vi "Pre Launch Init.vi"(11 "DIMActor in":refnum<class "DIMActor.lvclass">) -> (0 "error out":errorcluster, 3 "DIMActor out":refnum<class "DIMActor.lvclass">)   [LabVIEW 2012, in "DIMActor.lvlib" / "DIMActor.lvclass"]
doc: "Obtain references to DIM queue and notifier."
uses:
  DIMActor.lvclass
  DIMActor.lvclass/DIMActor.ctl
  <vilib>/ActorFramework/Actor/Actor.lvclass
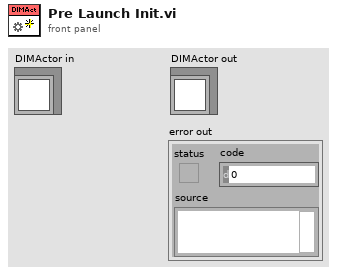
[diagram p1: front panel]
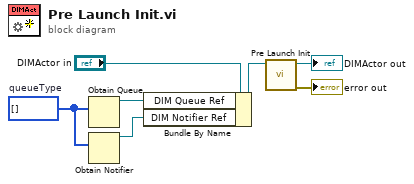
[diagram p0: block diagram]
diagram:
  w5 = i8[] []  # queueType
  n1 = Obtain Queue(element data type=w5) -> (queue out=w4:refnum<queue>)  [unwired: 4 in, 2 out]
  n2 = Obtain Notifier(notification data type=w5) -> (notifier out=w3:refnum<notifier>)  [unwired: 3 in, 2 out]
  n3 = Bundle By Name(cluster="DIMActor in", "DIM Queue Ref"=w4, "DIM Notifier Ref"=w3) -> (w1:refnum<class "DIMActor.lvclass">)
  n4 = call-parent "Pre Launch Init.vi"("Actor in"=w1) -> ("error out"=→"error out":errorcluster, "Actor out"=→"DIMActor out":refnum<class "DIMActor.lvclass">)  [unwired: 9 in]
